vi "ReadMotorEncoderUsingPdoRead.vi"(8 "error in (no error)":errorcluster, 11 "CANopen Session In":refnum<class "sbCANopenBaseClass.lvclass">) -> (2 "ReadValues":i32[](array[numeric]))   [LabVIEW 2024]
uses:
  <vilib>/addons/Maxon Motor/EPOS2 CANopen/CANopen/sbCANopenBaseClass.lvclass
  <vilib>/addons/Maxon Motor/EPOS2 CANopen/EPOS2 Support Files/Typedefs/EPOS2 PDO Object Data.ctl
  <vilib>/addons/Maxon Motor/EPOS2 CANopen/EPOS2 Library.lvlib
panel:
  out "error out 3":errorcluster
  out "Data 3":u8[](array[numeric])
  out "Position(qc)":i32
  out "error out 2":errorcluster
  out "Data 2":u8[](array[numeric])
  out "Veloxity(rpm)":i32
  out "Current(mA)":i32
  out "Data":u8[](array[numeric])
  out "error out":errorcluster
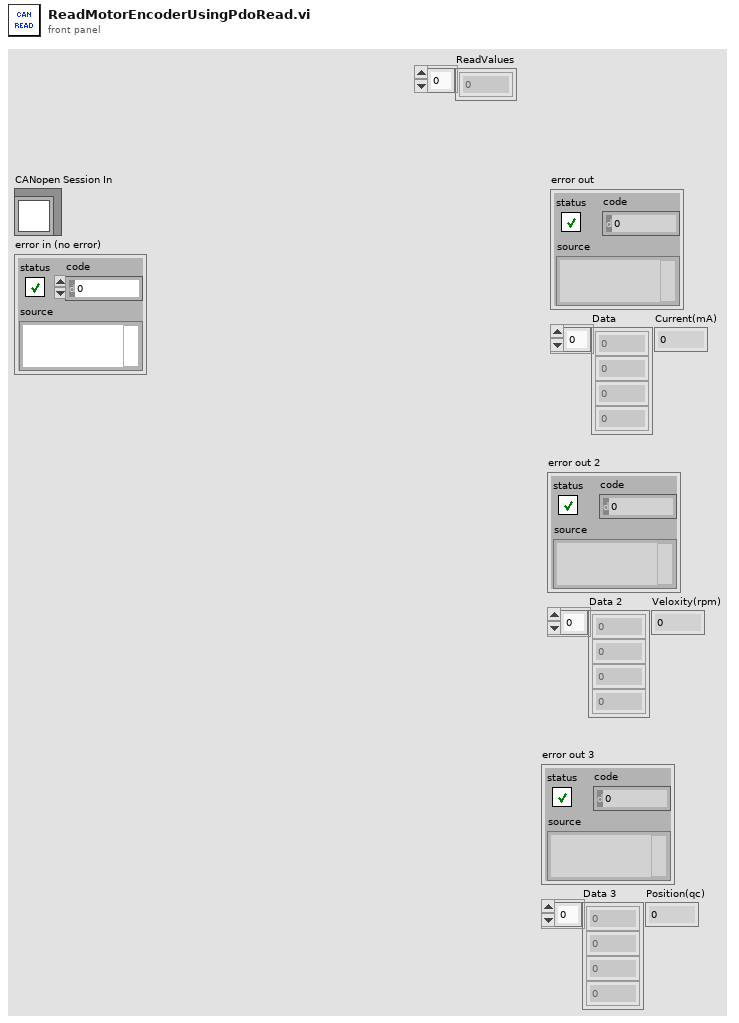
[diagram p1: front panel]
types:
  T1 = typedef "EPOS2 Library.lvlib/EPOS2 PDO Object Data.ctl" = cluster{"Index":u16, "Sub Index":u8, "Size":u8}
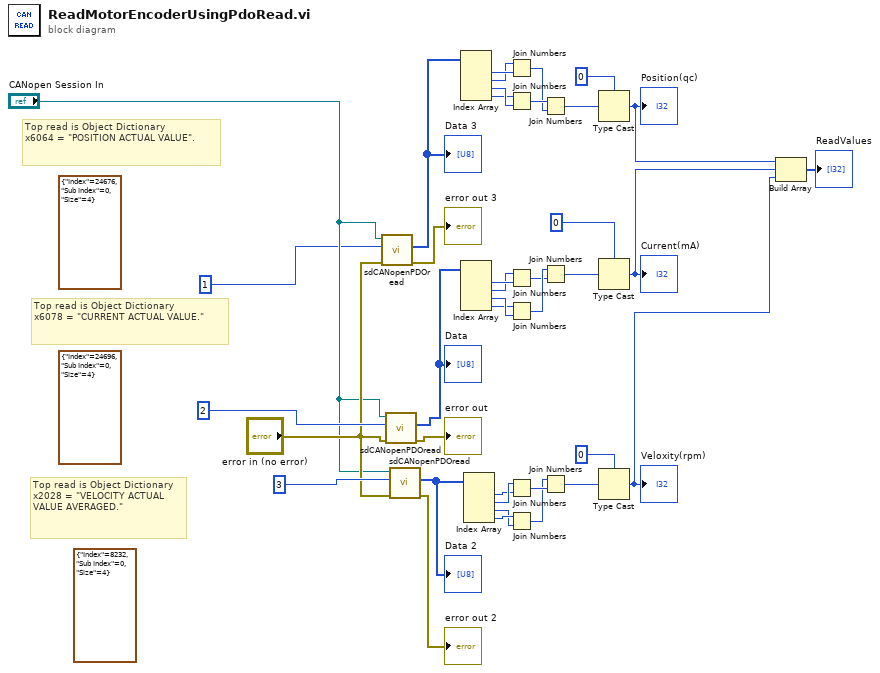
[diagram p0: block diagram]
diagram:
  (unwired) T1 {"Index"=24676, "Sub Index"=0, "Size"=4} ("PDO Object Data")
  (unwired) T1 {"Index"=8232, "Sub Index"=0, "Size"=4} ("PDO Object Data")
  (unwired) T1 {"Index"=24696, "Sub Index"=0, "Size"=4} ("PDO Object Data")
  # "Top read is Object Dictionary\nx2028 = \"VELOCITY ACTUAL\nVALUE AVERAGED.\""
  # "Top read is Object Dictionary\nx6078 = \"CURRENT ACTUAL VALUE.\""
  # "Top read is Object Dictionary\nx6064 = \"POSITION ACTUAL VALUE\"."
  n1 = call-dynamic "sdCANopenPDOread.vi"("error in (no error)"="error in (no error)", "PDO Number"=u8 1, "sbCANopenBaseClass in"="CANopen Session In") -> ("error out"=→"error out 3":errorcluster, "Data"=w5:u8[])  [unwired: 6 in, 1 out]
  "Data 3" <- w5
  n2 = call-dynamic "sdCANopenPDOread.vi"("error in (no error)"="error in (no error)", "PDO Number"=u8 2, "sbCANopenBaseClass in"="CANopen Session In") -> ("error out"=→"error out":errorcluster, "Data"=w7:u8[])  [unwired: 6 in, 1 out]
  "Data" <- w7
  n3 = call-dynamic "sdCANopenPDOread.vi"("error in (no error)"="error in (no error)", "PDO Number"=u8 3, "sbCANopenBaseClass in"="CANopen Session In") -> ("error out"=→"error out 2":errorcluster, "Data"=w8:u8[])  [unwired: 6 in, 1 out]
  "Data 2" <- w8
  n4 = Index Array(array=w5) -> (element #1=w22:u8, element #2=w21:u8, element #3=w20:u8, element #4=w19:u8)  [unwired: 4 in]
  n5 = Index Array(array=w7) -> (element #1=w38:u8, element #2=w37:u8, element #3=w36:u8, element #4=w35:u8)  [unwired: 4 in]
  n6 = Index Array(array=w8) -> (element #1=w27:u8, element #2=w28:u8, element #3=w29:u8, element #4=w30:u8)  [unwired: 4 in]
  n7 = Join Numbers(hi=w21, lo=w22) -> ((hi.lo)=w17:u16)
  n8 = Join Numbers(hi=w19, lo=w20) -> ((hi.lo)=w18:u16)
  n9 = Join Numbers(hi=w37, lo=w38) -> ((hi.lo)=w33:u16)
  n10 = Join Numbers(hi=w35, lo=w36) -> ((hi.lo)=w34:u16)
  n11 = Join Numbers(hi=w28, lo=w27) -> ((hi.lo)=w32:u16)
  n12 = Join Numbers(hi=w30, lo=w29) -> ((hi.lo)=w31:u16)
  n13 = Join Numbers(hi=w18, lo=w17) -> ((hi.lo)=w23:u32)
  n14 = Join Numbers(hi=w34, lo=w33) -> ((hi.lo)=w39:u32)
  n15 = Join Numbers(hi=w31, lo=w32) -> ((hi.lo)=w26:u32)
  n16 = Type Cast(type=0, x=w23) -> (*(type *) &x=w16:i32)
  "Position(qc)" <- w16
  n17 = Type Cast(type=0, x=w39) -> (*(type *) &x=w15:i32)
  "Current(mA)" <- w15
  n18 = Type Cast(type=0, x=w26) -> (*(type *) &x=w14:i32)
  "Veloxity(rpm)" <- w14
  n19 = Build Array(w16, w15, w14) -> (→"ReadValues":i32[])
